vi "Hopper Controller.vi"(8 "error in":errorcluster) -> ()   [LabVIEW 2025]
doc: "This VI executes continuously carrying out the current operation and responding to updates or new operations. It will often contain the timing or control code that is difficult to place directly in TeleOp. This VI generally opens all sensors and motors and isolates the rest of the robot code from knowing how the operations are carried out."
uses:
  <vilib>/Rock Robotics/WPI/Framework/Completion Status.ctl
  Hopper Setpoints.ctl
  Hopper Operations.ctl
  <vilib>/Rock Robotics/WPI/ThirdParty/REV Robotics/REVLib/Typedef/Spark MAX Idle Mode.ctl
  <vilib>/Rock Robotics/WPI/ThirdParty/REV Robotics/REVLib/Typedef/Spark MAX Control Type.ctl
  <vilib>/Rock Robotics/WPI/ThirdParty/REV Robotics/REVLib/SubVI/Public/SPARK Configure Power Current Limit.vi
  <vilib>/Rock Robotics/WPI/ThirdParty/REV Robotics/REVLib/SubVI/Public/SPARK Configure Basic Idle Mode.vi
  <vilib>/Rock Robotics/WPI/ThirdParty/REV Robotics/REVLib/SubVI/Public/SPARK Open Brushless.vi
  <vilib>/Rock Robotics/Network Tables/NT Write Boolean.vi
panel:
  in  "Interactive Values":T1
  out "Current\nCmd":string
  in  "Buttons":cluster{"Execute Cmd":bool, "Abort Cmd":bool}
  out "Command Timing":cluster{"Start Time (ms)":u32, "Iterations":i32}
  out "Status":T3
  # "Tip: It may be helpful to observe inputs and sensor values.\nYou may also want to display tuning or debugging controls."
  # "Interactive Command: You may fill in the settings for a command\nand schedule it with the Execute button. You can observe and abort\nany command while fine tuning the code for the controller."
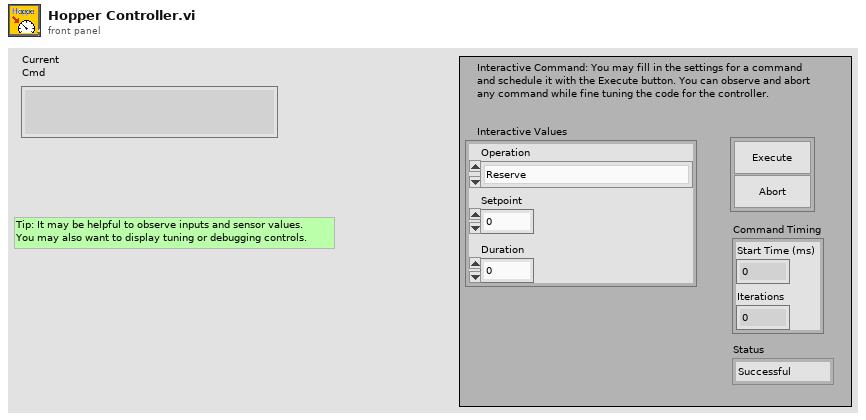
[diagram p1: front panel]
types:
  T1 = typedef "Hopper Setpoints.ctl" = cluster{"Operation":T2, "Setpoint":dbl, "Duration":dbl}
  T2 = typedef "Hopper Operations.ctl" = enum16{"Reserve", "Read Current", "Immediate"}
  T3 = typedef "Completion Status.ctl" = enum16{"Successful", "Aborted", "Incomplete"}
  T4 = typedef "Spark MAX Idle Mode.ctl" = enum16{"Coast", "Brake"}
  T5 = typedef "WPI_MotorControlDeviceRef.ctl" = cluster{"DeviceStatus":errorcluster, "Type":T6, "PWM":cluster{"PWM Channel":T7, "DeadBand":T8}, "CAN":cluster{"Device Number":u8, "SetOutput VI Ref":variant, "GetOutput VI Ref":variant, "Enable VI Ref":variant, "Disable VI Ref":variant, "Data":variant}, "Invert":bool, "DIO PWM":cluster{"PWM \"Enable\" Channel":T7, "DIOChannel":T9, "PWM Rate":dbl}}
  T6 = typedef "WPI_MotorControlType.ctl" = enum16{"PWM", "CAN", "DIO PWM"}
  T7 = typedef "FPGA_DIOPWMChannel.ctl" = enum8{"PWM 0", "PWM 1", "PWM 2", "PWM 3", "PWM 4", "PWM 5", "PWM 6", "PWM 7", "PWM 8", "PWM 9", "PWM MXP 0", "PWM MXP 1", "PWM MXP 2", "PWM MXP 3", "PWM MXP 4", "PWM MXP 5", "PWM MXP 6", "PWM MXP 7", "PWM MXP 8", "PWM MXP 9", "Invalid"}
  T8 = typedef "WPI_PWMDeadband.ctl" = cluster{"Name":string, "maxPositivePwm":i32, "minPositivePwm":i32, "centerPwm":i32, "maxNegativePwm":i32, "minNegativePwm":i32, "angularRange":u16}
  T9 = typedef "FPGA_DIOChannel.ctl" = enum8{"DIO 0", "DIO 1", "DIO 2", "DIO 3", "DIO 4", "DIO 5", "DIO 6", "DIO 7", "DIO 8", "DIO 9", "DIO MXP 0", "DIO MXP 1", "DIO MXP 2", "DIO MXP 3", "DIO MXP 4", "DIO MXP 5", "DIO MXP 6", "DIO MXP 7", "DIO MXP 8", "DIO MXP 9", "DIO MXP 10", "DIO MXP 11", "DIO MXP 12", "DIO MXP 13", "DIO MXP 14", "DIO MXP 15", "SPI Port CS1", "SPI Port CS2", "SPI Port CS3", "SPI Port MISO", "SPI Port MOSI", "Invalid"}
  T10 = typedef "Command Status Info.ctl" = cluster{"Name":string, "Status":T3, "notifier out":T11}
  T11 = typedef "Completion Notifier.ctl" = refnum<notifier>
  T12 = cluster{"Current Command":T1, "Command Timing":cluster{"Start Time (ms)":u32, "Iterations":i32}, "Command Arguments":cluster{"Command Info":T10, "Description":string, "Default Command":T1, "queue out":refnum<queue>, "Subsystem Name":string}}
  T13 = typedef "Spark MAX Control Type.ctl" = enum16{"Percent VBus", "Voltage", "Velocity", "Position", "Smart Motion", "Current", "Smart Velocity", "MAXMotion Position", "MAXMotion Velocity"}
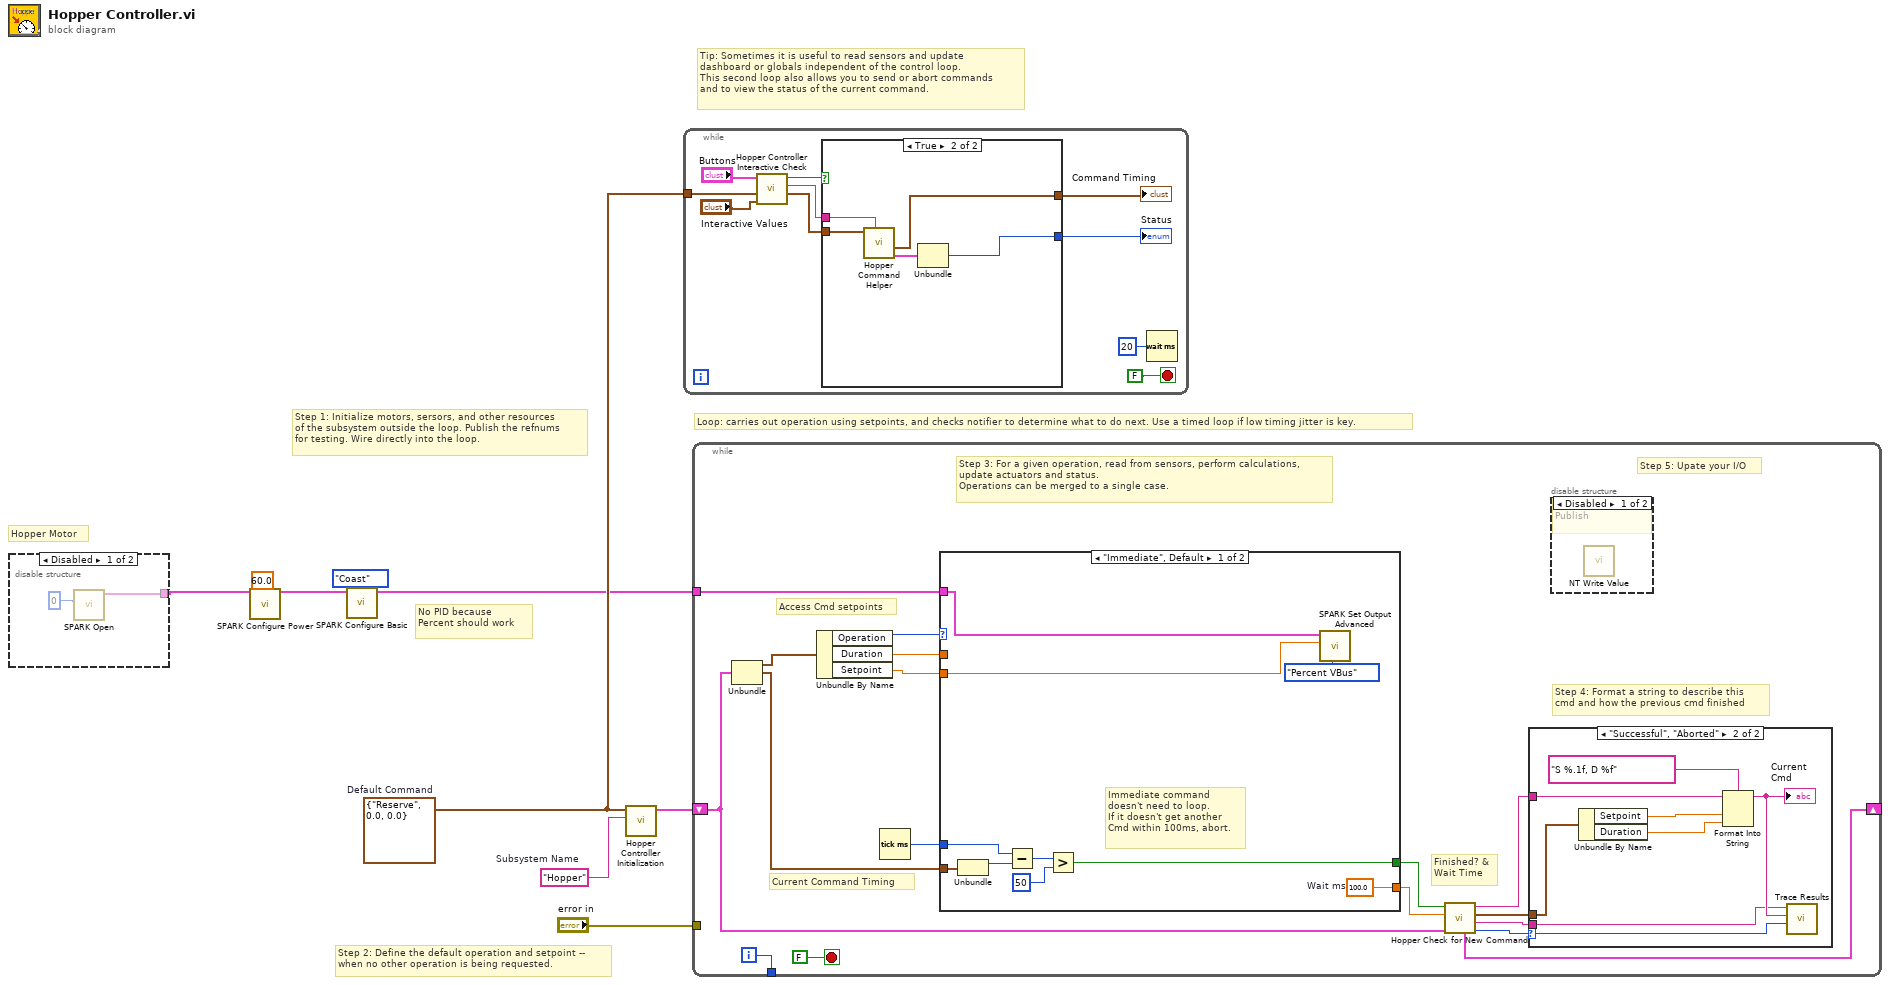
[diagram p0: block diagram]
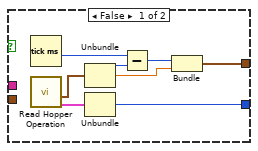
[diagram p3: hidden frame]
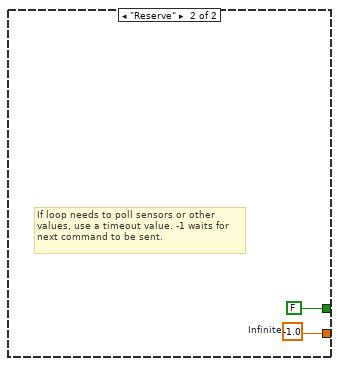
[diagram p6: hidden frame]
diagram:
  w4 = T1 {"Operation"=enum."Reserve", "Setpoint"=0.0, "Duration"=0.0}  # Default Command
  w5 = "Hopper"  # Subsystem Name
  # "No PID because Percent should work"
  # "Hopper Motor"
  # "Tip: Sometimes it is useful to read sensors and update\ndashboard or globals independent of the control loop.\nThis second loop also allows you to send or abort commands\nand to view the status of the current command."
  # "Step 2: Define the default operation and setpoint --\nwhen no other operation is being requested."
  # "Step 1: Initialize motors, sersors, and other resources\nof the subsystem outside the loop. Publish the refnums\nfor testing. Wire directly into the loop."
  # "Loop: carries out operation using setpoints, and checks notifier to determine what to do next. Use a timed loop if low timing jitter is key."
  n1 = disable-structure shown="Disabled" {
    disable-tunnel: [w8 _] -> w1
    frame Disabled {
      n2 = call-poly <vilib>:"SPARK Open.vi"("Device Number"=u8 0) -> ("MotorControlDeviceRef"=w8:T5)  [unwired: 9 in, 1 out]
    }
    frame Enabled {
    }
  }
  n3 = call-poly <vilib>:"SPARK Configure Power.vi"("Current Limit A (100)"=sgl 60.0, "MotorControlDeviceRef in"=w1) -> ()  [unwired: 8 in, 2 out]
  n4 = call-poly <vilib>:"SPARK Configure Basic.vi"("Idle Mode"=Spark_MAX_Idle_Mode."Coast", "MotorControlDeviceRef in"=w1) -> ()  [unwired: 8 in, 2 out]
  n5 = call "Hopper Controller Initialization.vi"("Subsystem Name"=w5, "Default Command"=w4) -> ("Current Command"=w6:T12)  [unwired: 9 in]
  n6 = while {
    tunnel: w4 -> [w16]
    stop <- FALSE stop-if-true
    n7 = call "Hopper Controller Interactive Check.vi"("Interactive Command in"="Interactive Values", "Default Command"=w16, "Buttons"="Buttons") -> ("Interactive Command out"=w13:T1, "Trace String"=w14:string, "Schedule"=w15:bool)  [unwired: 6 in]
    n8 = case shown="True" w15 {
      tunnel: [w27 w32] -> w12
      tunnel: w13 -> [_ w30]
      tunnel: [w23 w28] -> w11
      tunnel: w14 -> [_ w31]
      frame False {
        n9 = Tick Count (ms)() -> (millisecond timer value=w22:u32)
        n10 = call "Read Hopper Operation.vi"() -> ("Command Info"=w20:T10, "SubSystem Data"=w21:T1)  [unwired: 9 in, 1 out]
        n11 = Unbundle(w21) -> ("Operation"=w26:T2, "Setpoint"=w24:dbl)  [unwired: 1 out]
        n12 = Unbundle(w20) -> ("Status"=w27:T3)  [unwired: 2 out]
        n13 = Subtract(x=w22, y=w26) -> (x-y=w25:u32)
        n14 = Bundle(w25, "Setpoint"=w24) -> (w23:cluster{u32, "Setpoint":dbl})  [unwired: 1 in]
      }
      frame True {
        n15 = call "Hopper Command Helper.vi"("Description"=w31, "SubSystem Data"=w30) -> ("Command Info Out"=w29:T10, "Command Timing"=w28:cluster{"Start Time (ms)":u32, "Iterations":i32})  [unwired: 7 in, 1 out]
        n16 = Unbundle(w29) -> ("Status"=w32:T3)  [unwired: 2 out]
      }
    }
    "Status" <- w12
    "Command Timing" <- w11
    n17 = Wait (ms)(milliseconds to wait=u32 20) -> ()  [unwired: 1 out]
  }
  n18 = while {
    shift-right: [w41] -> _
    shift-left: w6 -> [w34]
    tunnel: [w48] -> _
    tunnel: "error in" -> [_]
    tunnel: w1 -> [w33]
    i -> [w48]
    stop <- FALSE stop-if-true
    # "Step 5: Upate your I/O"
    # "Step 4: Format a string to describe this\ncmd and how the previous cmd finished"
    # "Current Command Timing"
    # "Access Cmd setpoints"
    # "Finished? &\nWait Time"
    # "Step 3: For a given operation, read from sensors, perform calculations,\nupdate actuators and status.\nOperations can be merged to a single case."
    n19 = Unbundle(w34) -> ("Current Command"=w47:T1, "Command Timing"=w43:cluster{"Start Time (ms)":u32, "Iterations":i32})  [unwired: 1 out]
    n20 = Unbundle By Name(w47) -> ("Operation"=w46:T2, "Duration"=w45:dbl, "Setpoint"=w42:dbl)
    n21 = Tick Count (ms)() -> (millisecond timer value=w44:u32)
    n22 = case shown="\"Immediate\", Default" w46 {
      tunnel: [w67 w69] -> w39
      tunnel: [w61 FALSE ("ignore previous (F)")] -> w40
      tunnel: w43 -> [w63 _]
      tunnel: w45 -> [_ _]
      tunnel: w44 -> [w62 _]
      tunnel: w42 -> [w58 _]
      tunnel: w33 -> [w59 _]
      frame "Immediate", Default {
        w67 = 100.0  # Wait ms
        # "Immediate command\ndoesn't need to loop.\nIf it doesn't get another\nCmd within 100ms, abort."
        n23 = Unbundle(w63) -> ("Start Time (ms)"=w66:u32)  [unwired: 1 out]
        n24 = Subtract(x=w62, y=w66) -> (x-y=w65:u32)
        n25 = Greater?(x=w65, y=u8 50 ("Left Motor")) -> (0:w61:bool)
        n26 = call <vilib>:"SPARK Set Output Advanced.vi"("Control Mode"=Spark_MAX_Control_Type."Percent VBus", "Setpoint"=w58, "MotorControlDevRef"=w59) -> ()  [unwired: 7 in, 2 out]
      }
      frame "Reserve" {
        w69 = -1.0  # Infinite
        # "If loop needs to poll sensors or other\nvalues, use a timeout value. -1 waits for\nnext command to be sent."
      }
    }
    n27 = call "Hopper Check for New Command.vi"("Current Command"=w34, "Wait time (ms)"=w39, "Finished?"=w40) -> ("Completion"=w35:T3, "Subsystem Name"=w36:string, "Current Command"=w37:T1, "Initial Trace String"=w38:string, "NextCommand"=w41:T12)  [unwired: 4 in]
    n28 = case shown="\"Successful\", \"Aborted\"" w35 {
      selector: w35 -> [_ w57]
      tunnel: w38 -> [_ w53]
      tunnel: w37 -> [_ w54]
      tunnel: w36 -> [_ w50]
      frame "Incomplete", Default {
        # "Continuing current command"
      }
      frame "Successful", "Aborted" {
        # "Report and setup for next command"
        n29 = Unbundle By Name(w54) -> ("Setpoint"=w56:dbl, "Duration"=w51:dbl)
        n30 = Format Into String(format string="S %.1f, D %f", initial string=w53, w56, w51) -> (resulting string=w52:string)  [unwired: 1 in, 1 out]
        "Current\nCmd" <- w52
        n31 = call <vilib>:"Trace Results.vi"("Status of previous command"=w57, "Description"=w52, "Subsystem"=w50) -> ()  [unwired: 9 in]
      }
    }
    n32 = disable-structure shown="Disabled" {
      frame Disabled {
        # "Publish"
        n33 = call-poly <vilib>:"NT Write Value.vi"() -> ()  [unwired: 11 in, 1 out]
      }
      frame Enabled {
      }
    }
  }
